vi "Init.vi"(3 "Container State":T4, 4 "Previous State":variant, 5 "Previous Version":T3) -> (2 "Current State":T1)   [LabVIEW 2017, in "3D Mesh.xctl"]
uses:
  <vilib>/Math Plots/3D Math Plots/3D Mesh/3D Mesh XCtrl/3D Mesh.xctl
  <vilib>/Math Plots/3D Math Plots/3D Mesh/3D Mesh XCtrl/State.ctl
  <vilib>/Math Plots/3D Math Plots/3D Mesh/3D Mesh/3D Mesh.lvclass
  <vilib>/Math Plots/3D Math Plots/3D Plot/Action String/3DMathPlot Ctrl Act Queue.ctl
  <vilib>/Math Plots/3D Math Plots/3D Plot/Action String/3DMathPlot Ctrl Act Cluster.ctl
  <vilib>/Math Plots/3D Math Plots/3D Plot/Action String/3DMathPlot State Class.ctl
  <vilib>/_xctls/Container State.ctl
  <vilib>/_xctls/Version.ctl
  <vilib>/_xctls/XControlSupport.lvlib
panel:
  in  "Default Indicator State":T1={"3D Mesh.lvclass"=refnum, "Control Ref Queue"=refnum, "Main Frame Color"=12369084, "Ramp Palette Color"=12369084, "Projection Palette Color"=12369084}
  in  "Default Control State":T1={"3D Mesh.lvclass"=refnum, "Control Ref Queue"=refnum, "Main Frame Color"=12369084, "Ramp Palette Color"=12369084, "Projection Palette Color"=12369084}
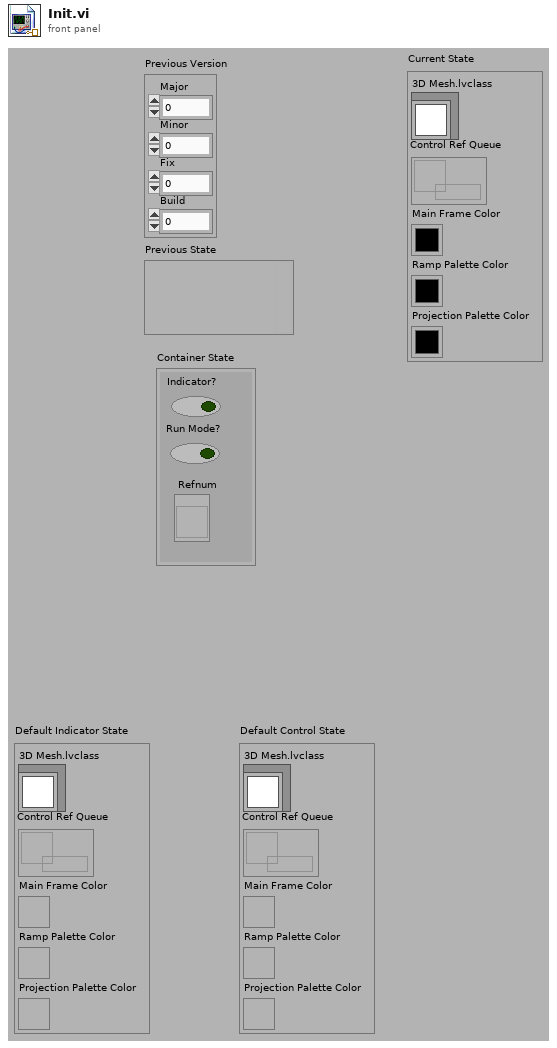
[diagram p1: front panel]
types:
  T1 = typedef "3D Mesh.xctl/State.ctl" = cluster{"3D Mesh.lvclass":refnum<class "3D Mesh.lvclass">, "Control Ref Queue":T2, "Main Frame Color":u32, "Ramp Palette Color":u32, "Projection Palette Color":u32}
  T2 = typedef "3DMathPlot Ctrl Act Queue.ctl" = refnum<queue>
  T3 = typedef "XControlSupport.lvlib/Version.ctl" = cluster{"Major":u16, "Minor":u16, "Fix":u16, "Build":u16}
  T4 = typedef "XControlSupport.lvlib/Container State.ctl" = cluster{"Indicator?":bool, "Run Mode?":bool, " Refnum":refnum<vi>}
  T5 = typedef "3DMathPlot Ctrl Act Cluster.ctl" = cluster{"3D Picture Control":refnum<vi>, "Render Window Refnum":refnum<vi>, "XY Graph":refnum<vi>, "Intensity Graph":refnum<vi>, "Color Legend Palette":refnum<vi>, "Projection Palette":refnum<vi>, "XControl  Ref":refnum<vi>, "Facade Ref":refnum<vi>, "Export Image Ref":refnum<vi>, "Clear Data Flag":bool, "Display State Change Class":T6}
  T6 = typedef "3DMathPlot State Class.ctl" = enum16{"Update All Objects (Undo)", "Update Light Object Only", "Update Axis Object Only", "Update Plot Object Only", "Update Cursor Object Only", "Update Axis Plot Cursor Objects", "No Update"}
  T7 = cluster{"3D Mesh.lvclass":refnum<class "3D Mesh.lvclass">, "Control Ref Queue":T2}
  T8 = cluster{"3D Mesh.lvclass":refnum<class "3D Mesh.lvclass">, "Control Ref Queue":T2, "Frame Color":u32, "Frame Color":u32, "Frame Color":u32}
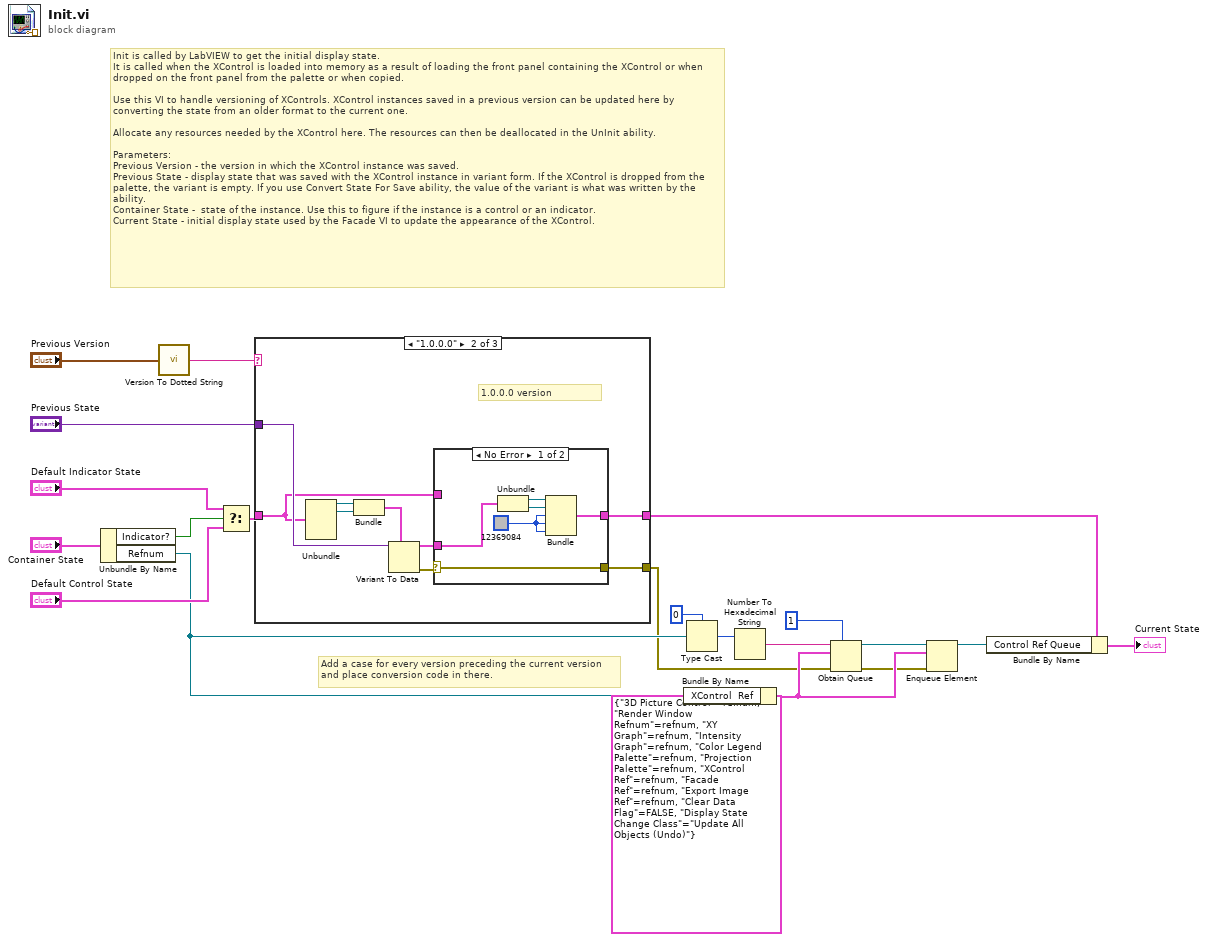
[diagram p0: block diagram]
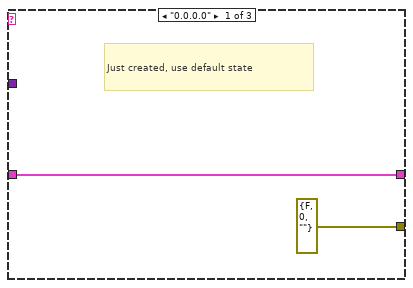
[diagram p2: hidden frame]
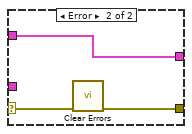
[diagram p3: hidden frame]
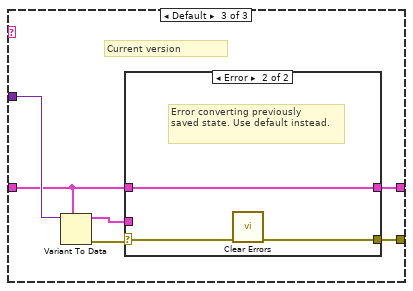
[diagram p4: hidden frame]
diagram:
  # "Init is called by LabVIEW to get the initial display state.\nIt is called when the XControl is loaded into memory as a result of loading the front panel containing the XControl or when dropped on the front panel from the palette or when copied.\n\nUse this VI to handle versioning of XControls. XControl instances saved in a previous version can be updated here by converting the state from an older format to the current one.\n\nAllocate any resources needed by the XControl here. The resources can then be deallocated in the UnInit ability.\n\nParameters:\nPrevious Version - the version in which the XControl instance was saved.\nPrevious State - display state that was saved with the XControl instance in variant form. If the XControl is dropped from the palette, the variant is empty. If you use Convert State For Save ability, the value of the variant is what was written by the ability. \nContainer State -  state of the instance. Use this to figure if the instance is a control or an indicator.\nCurrent State - initial display state used by the Facade VI to update the appearance of the XControl."
  # "Add a case for every version preceding the current version and place conversion code in there."
  n1 = Unbundle By Name("Container State") -> ("Indicator?"=w17:bool, "Refnum"=w4:refnum<vi>)
  n2 = call <vilib>:"Version To Dotted String.vi"("Version"="Previous Version") -> ("String Version"=w14:string)
  n3 = Select(t="Default Indicator State", s=w17, f="Default Control State") -> (s? t:f=w16:T1)
  n4 = case shown="\"1.0.0.0\"" w14 {
    tunnel: "Previous State" -> [_ w27 w47]
    tunnel: [w23 w25 w43] -> w9
    tunnel: w16 -> [w23 w26 w44]
    tunnel: [errorcluster {"status"=FALSE, "code"=0, "source"=""} ("error IO") w24 w42] -> w2
    frame "0.0.0.0" {
      # "Just created, use default state"
    }
    frame "1.0.0.0" {
      # "1.0.0.0 version"
      n5 = Unbundle(w26) -> ("3D Mesh.lvclass"=w31:refnum<class "3D Mesh.lvclass">, "Control Ref Queue"=w32:T2)  [unwired: 3 out]
      n6 = Bundle("3D Mesh.lvclass"=w31, "Control Ref Queue"=w32) -> (w30:T7)  [unwired: 1 in]
      n7 = Variant To Data(type=w30, Variant=w27) -> (data=w29:T7, error out=w28:errorcluster)  [unwired: 1 in]
      n8 = case shown="No Error" w28 {
        selector: w28 -> [w38 w40]
        tunnel: w29 -> [w36 _]
        tunnel: [w34 w41] -> w25
        tunnel: w26 -> [_ w41]
        tunnel: [w38 w39] -> w24
        frame No Error {
          w33 = u32 12369084 ("Frame Color")
          n9 = Unbundle(w36) -> ("3D Mesh.lvclass"=w37:refnum<class "3D Mesh.lvclass">, "Control Ref Queue"=w35:T2)
          n10 = Bundle("3D Mesh.lvclass"=w37, "Control Ref Queue"=w35, "Frame Color"=w33, "Frame Color"=w33, "Frame Color"=w33) -> (w34:T8)  [unwired: 1 in]
        }
        frame Error {
          n11 = call <vilib>:"Clear Errors.vi"("error in (no error)"=w40) -> ("error out"=w39:errorcluster)  [unwired: 1 in, 5 out]
        }
      }
    }
    frame Default {
      # "Current version"
      n12 = Variant To Data(type=w44, Variant=w47) -> (data=w45:T1, error out=w46:errorcluster)  [unwired: 1 in]
      n13 = case shown="Error" w46 {
        selector: w46 -> [w49 w51]
        tunnel: w45 -> [w48 _]
        tunnel: [w48 w52] -> w43
        tunnel: w44 -> [_ w52]
        tunnel: [w49 w50] -> w42
        frame No Error {
        }
        frame Error {
          # "Error converting previously \nsaved state. Use default instead."
          n14 = call <vilib>:"Clear Errors.vi"("error in (no error)"=w51) -> ("error out"=w50:errorcluster)  [unwired: 1 in, 5 out]
        }
      }
    }
  }
  n15 = Bundle By Name(cluster=T5 {"3D Picture Control"=refnum, "Render Window Refnum"=refnum, "XY Graph"=refnum, "Intensity Graph"=refnum, "Color Legend Palette"=refnum, "Projection Palette"=refnum, "XControl  Ref"=refnum, "Facade Ref"=refnum, "Export Image Ref"=refnum, "Clear Data Flag"=FALSE, "Display State Change Class"=enum."Update All Objects (Undo)"} ("Control Ref Cluster"), "XControl  Ref"=w4) -> (w3:T5)
  n16 = Type Cast(type=u64 0, x=w4) -> (*(type *) &x=w13:u64)
  n17 = Number To Hexadecimal String(2:w13) -> (0:w11:string)  [unwired: 1 out]
  n18 = Obtain Queue(max queue size (-1, unlimited)=1, name (unnamed)=w11, element data type=w3, error in (no error)=w2) -> (queue out=w7:refnum<queue>, error out=w1:errorcluster)  [unwired: 1 in, 1 out]
  n19 = Enqueue Element(queue=w7, element=w3, error in (no error)=w1) -> (queue out=w6:refnum<queue>)  [unwired: 3 out]
  n20 = Bundle By Name(cluster=w9, "Control Ref Queue"=w6) -> (→"Current State":T1)
